vi "Ini_SetOutput.vi"(8 "error in (no error)":errorcluster, 11 "2410C-64 in":refnum<class "2410C-64.lvclass">) -> (0 "error out":errorcluster, 3 "2410C-64 out":refnum<class "2410C-64.lvclass">)   [LabVIEW 2019, in "2410C-64.lvclass"]
uses:
  2410C-64.lvclass
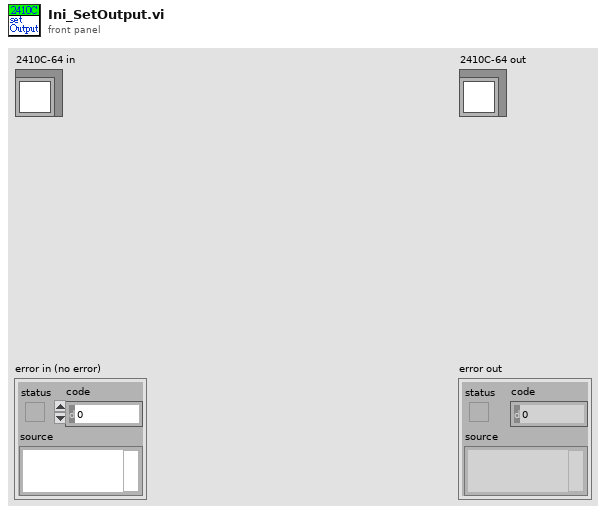
[diagram p1: front panel]
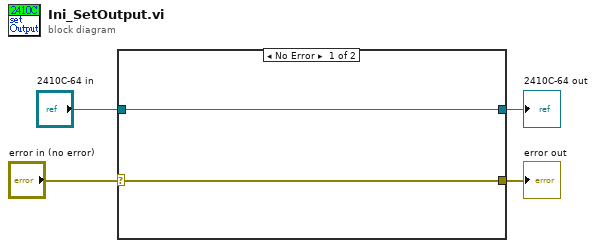
[diagram p0: block diagram]
diagram:
  n1 = case shown="No Error" "error in (no error)" {
    selector: "error in (no error)" -> [w5 w7]
    tunnel: "2410C-64 in" -> [w6 w8]
    tunnel: [w6 w8] -> w2
    tunnel: [w5 w7] -> w1
    frame No Error {
    }
    frame Error {
    }
  }
  "error out" <- w1
  "2410C-64 out" <- w2
